vi "Trajectory Loading v2.vi"(6 "PID Cluster":T6={"L1 to L4 PID Cluster"={"L1 PID Gains"={"Kp"=0.005, "Kd"=0.5, "Ki"=0.0005}, "L2 PID Gains"={"Kp"=0.01, "Kd"=1.0, "Ki"=0.005}, "L3 PID Gains"={"Kp"=0.05, "Kd"=1.0, "Ki"=0.0005}, "L4 PID Gains"={"Kp"=0.1, "Kd"=0.1, "Ki"=0.0005}}, "Stage PID Cluster"={"Stage Z PID"={"Kp"=0.0005, "Kd"=0.001, "Ki"=0.0}, "Stage Y PID"={"Kp"=0.0003, "Kd"=0.01, "Ki"=0.0}, "Stage X PID"={"Kp"=0.0003, "Kd"=0.01, "Ki"=0.0}}, "OCT Z PID Gains"={"Kp"=0.0003, "Kd"=0.0001, "Ki"=0.01}}, 7 "Robot In":i32, 8 "error in":errorcluster, 10 "Prev Posit Cluster":T5={"Prev L1 to L4 Posit"=[-0.5319, -0.035669172703475985, -2.0566170657346783, 0.9099264705882353], "Prev Stage Posit"=[6.002553885707208, 5.996566124542428, 5.995469940427586], "Prev OCT Z Posit"=-0.0}, 11 "FPGA VI Reference In":refnum<k20>) -> (0 "Eye Model Cluster":T3={"X Grid"=[], "Y Grid"=[], "Za_true Surf"=[], "Iris Center"=[0.0, 5.0, 0.0], "Zp_true Surf"=[], "Pinv"=[[1.0, 0.0], [0.0, 1.0]], "za_true"=0.0, "za_work"=0.0, "zp_work"=0.0, "zp_true"=0.0}, 1 "Trajectory Cluster":T1, 2 "Last Posit Cluster":T4={"Last L1 to L4 Posit"=[0.0, 0.0, 0.0, 0.0], "Last Stage Posit"=[6.0, 6.0, 6.0], "Last OCT Z Posit"=0.0}, 3 "FPGA VI Reference Out":refnum<k20>, 4 "error out":errorcluster, 5 "First Trk Pt":dbl[](array[numeric]))   [LabVIEW 2016]
uses:
  Subsystems/Global Variables.vi
  <vilib>/Platform/TimedLoop/XDataNode/wakeup.ctl
  <vilib>/Platform/TimedLoop/XDataNode/XDNodeRunTimeDep.lvlib
  <vilib>/Platform/TimedLoop/XDataNode/nitl_modes.ctl
  <vilib>/Platform/TimedLoop/XDataNode/timing_clust.ctl
  <vilib>/platform/TimedLoop/XDataNode/XDataNode.xnode
  <vilib>/Analysis/Matrix/Datatypes/RealMatrix.ctl
  <vilib>/Analysis/Matrix/NI_Matrix.lvlib
panel:
  out "In Servo Loop":bool
  out "Loading Finished":bool
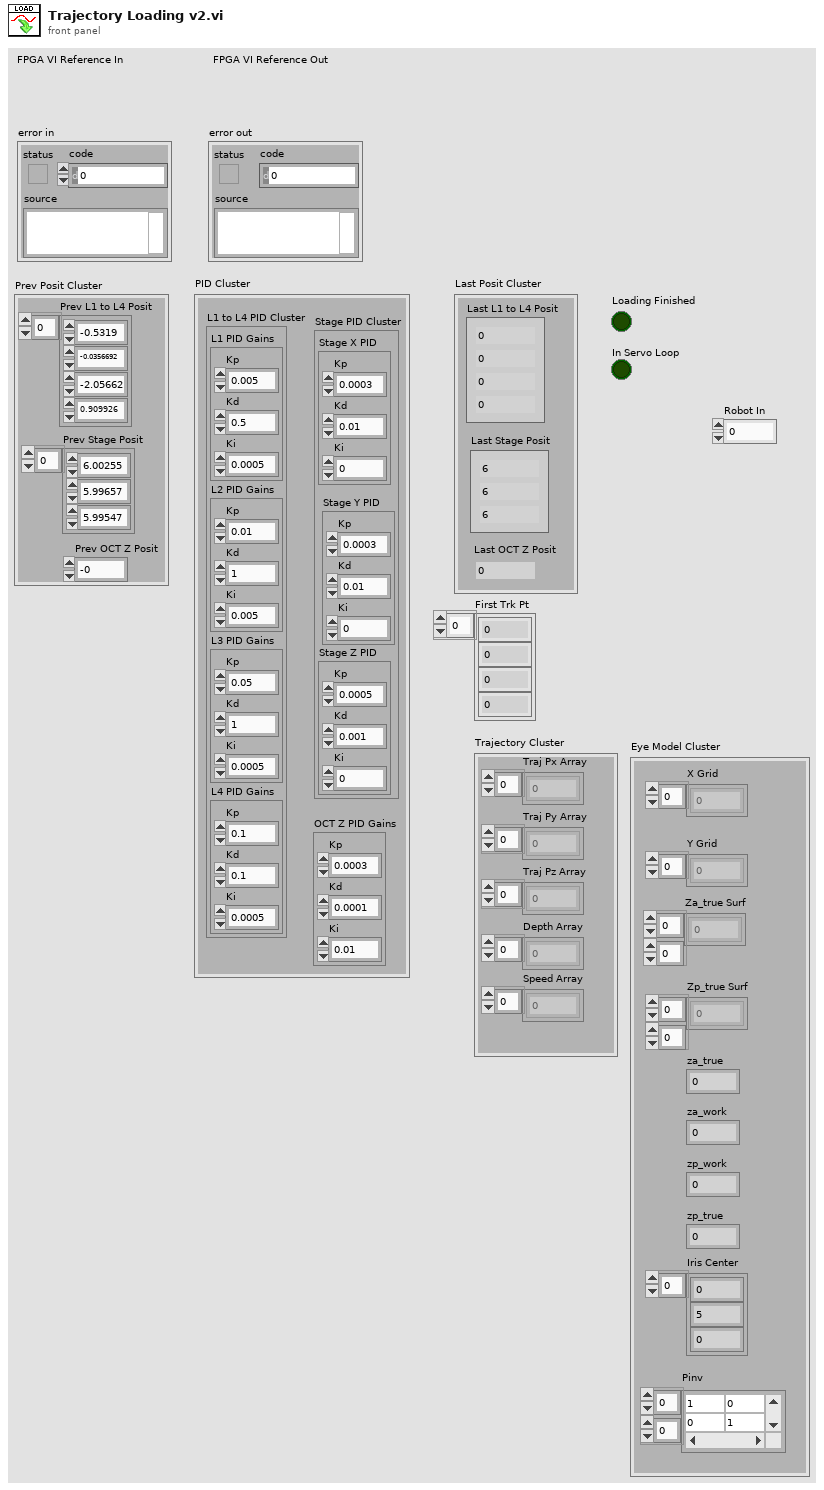
[diagram p1: front panel]
types:
  T1 = cluster{"Traj Px Array":dbl[], "Traj Py Array":dbl[], "Traj Pz Array":dbl[], "Speed Array":dbl[], "Depth Array":dbl[]}
  T2 = typedef "NI_Matrix.lvlib/RealMatrix.ctl" = dbl[][]
  T3 = cluster{"X Grid":dbl[], "Y Grid":dbl[], "Za_true Surf":dbl[][], "Iris Center":dbl[], "Zp_true Surf":dbl[][], "Pinv":T2, "za_true":dbl, "za_work":dbl, "zp_work":dbl, "zp_true":dbl}
  T4 = cluster{"Last L1 to L4 Posit":dbl[], "Last Stage Posit":dbl[], "Last OCT Z Posit":dbl}
  T5 = cluster{"Prev L1 to L4 Posit":dbl[], "Prev Stage Posit":dbl[], "Prev OCT Z Posit":dbl}
  T6 = cluster{"L1 to L4 PID Cluster":cluster{"L1 PID Gains":cluster{"Kp":dbl, "Kd":dbl, "Ki":dbl}, "L2 PID Gains":cluster{"Kp":dbl, "Kd":dbl, "Ki":dbl}, "L3 PID Gains":cluster{"Kp":dbl, "Kd":dbl, "Ki":dbl}, "L4 PID Gains":cluster{"Kp":dbl, "Kd":dbl, "Ki":dbl}}, "Stage PID Cluster":cluster{"Stage Z PID":cluster{"Kp":dbl, "Kd":dbl, "Ki":dbl}, "Stage Y PID":cluster{"Kp":dbl, "Kd":dbl, "Ki":dbl}, "Stage X PID":cluster{"Kp":dbl, "Kd":dbl, "Ki":dbl}}, "OCT Z PID Gains":cluster{"Kp":dbl, "Kd":dbl, "Ki":dbl}}
  T7 = typedef "XDNodeRunTimeDep.lvlib/timing_clust.ctl" = cluster{"Expected End [f-1]":u64, "Actual End [f-1]":u64, "Finished Late? [f-1]":bool, "Expected End [i-1]":u64, "Actual End [i-1]":u64, "Finished Late? [i-1]":bool, "Expected Start [i]":u64, "Actual Start [i]":u64, "Expected Start [f]":u64, "Actual Start [f]":u64, "Source Name":string, "Structure Name":string, "Period":i64, "Deadline":i64, "Offset":i64, "Start":i64, "Priority":i32, "Timeout":i32, "Mode":T8, "Wakeup Reason":T9, "Error":errorcluster, "Source Type":string, "Secondary Source Type":string, "Global End Time":u64, "Global Start Time":u64, "Frame Duration":u64, "Iteration Duration":u64, "Assigned CPU":i32, "I/O Scan Engine Mode":u32}
  T8 = typedef "XDNodeRunTimeDep.lvlib/nitl_modes.ctl" = enum32{"No Change", "Process missed periods, maintain original phase", "Discard missed periods, maintain original phase", "Process missed periods, ignore original phase", "Discard missed periods, ignore original phase"}
  T9 = typedef "XDNodeRunTimeDep.lvlib/wakeup.ctl" = enum32{"Normal", "Aborted", "Asynchronous wakeup", "Timing source error", "Timed loop error", "Timeout"}
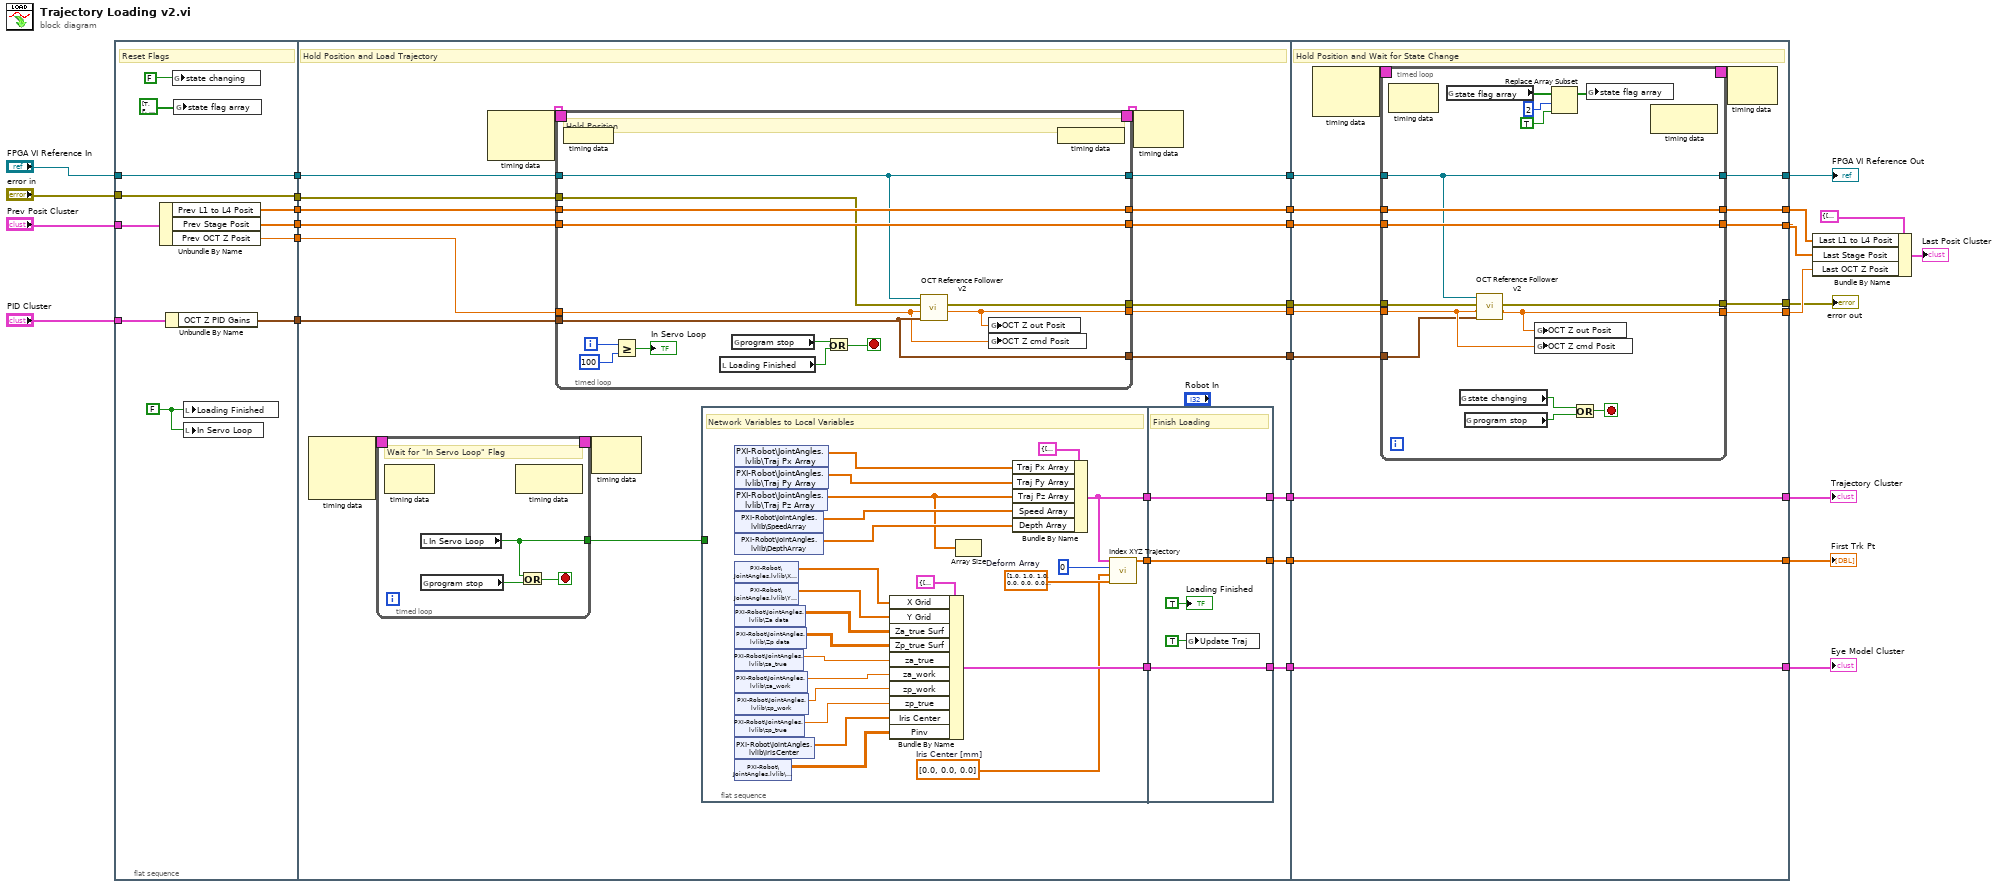
[diagram p0: block diagram]
diagram:
  n1 = flat-sequence {
    tunnel: [w38] -> w29
    tunnel: "FPGA VI Reference In" -> [w38]
    tunnel: [w37] -> w27
    tunnel: "error in" -> [w37]
    tunnel: "Prev Posit Cluster" -> [w36]
    tunnel: "PID Cluster" -> [w35]
    tunnel: [w34] -> w23
    tunnel: [w33] -> w22
    tunnel: [w32] -> w21
    tunnel: [w30] -> w20
    tunnel: w29 -> [w50]
    tunnel: w27 -> [w47]
    tunnel: w23 -> [w49]
    tunnel: w22 -> [w46]
    tunnel: w21 -> [w45]
    tunnel: w20 -> [w48]
    tunnel: [w63] -> w11
    tunnel: [w62] -> w10
    tunnel: [w61] -> w9
    tunnel: [w60] -> w8
    tunnel: [w59] -> w7
    tunnel: [w58] -> w6
    tunnel: [w41] -> w5
    tunnel: [w44] -> w4
    tunnel: [w42] -> w3
    tunnel: w11 -> [w130]
    tunnel: [w129] -> w1
    tunnel: w10 -> [w128]
    tunnel: w9 -> [w127]
    tunnel: w8 -> [w126]
    tunnel: w7 -> [w125]
    tunnel: [w124] -> w18
    tunnel: [w123] -> w17
    tunnel: [w122] -> w16
    tunnel: [w121] -> w14
    tunnel: [w118] -> w12
    tunnel: w6 -> [w120]
    tunnel: [w120] -> w13
    tunnel: w5 -> [w119]
    tunnel: w4 -> [w118]
    tunnel: [w117] -> w2
    tunnel: w3 -> [w117]
    frame #0 {
      w31 = FALSE ("Loading Finished")
      # "Reset Flags"
      n2 = Unbundle By Name(w36) -> ("Prev L1 to L4 Posit"=w34:dbl[], "Prev Stage Posit"=w33:dbl[], "Prev OCT Z Posit"=w32:dbl)
      n3 = Unbundle By Name(w35) -> ("OCT Z PID Gains"=w30:cluster{"Kp":dbl, "Kd":dbl, "Ki":dbl})
      n4 = global write "Global Variables.vi" "state changing"(FALSE ("state changing")) -> ()
      n5 = global write "Global Variables.vi" "state flag array"(bool[] [TRUE, FALSE, FALSE, FALSE, FALSE, FALSE, FALSE, FALSE, FALSE] ("state flag array")) -> ()
      n6 = local write "Loading Finished"(w31) -> ()
      n7 = local write "In Servo Loop"(w31) -> ()
    }
    frame #1 {
      # "Hold Position and Load Trajectory"
      n8 = node-c288() -> (w53:T7)  [unwired: 3 in]
      n9 = timed-loop {
        timing: w53 -> [_]
        timing-out: [_] -> w52
        tunnel: [w65] -> w51
        stop <- w66 stop-if-true
        # "Wait for \"In Servo Loop\" Flag"
        n10 = node-c288() -> ()  [unwired: 1 in, 1 out]
        n11 = local read "In Servo Loop"() -> (w65:bool)
        n12 = global read "Global Variables.vi" "program stop"() -> (w64:bool)
        n13 = node-c288() -> ()  [unwired: 1 in, 1 out]
        n14 = Or(x=w65, y=w64) -> (x .or. y?=w66:bool)
      }
      n15 = node-c288() -> (w57:T7)  [unwired: 2 in]
      n16 = timed-loop {
        timing: w57 -> [_]
        timing-out: [_] -> w56
        tunnel: w49 -> [w105]
        tunnel: w46 -> [w106]
        tunnel: w47 -> [w102]
        tunnel: w50 -> [w101]
        tunnel: w45 -> [w103]
        tunnel: w48 -> [w104]
        tunnel: [w105] -> w62
        tunnel: [w106] -> w61
        tunnel: [w99] -> w60
        tunnel: [w101] -> w63
        tunnel: [w100] -> w41
        tunnel: [w104] -> w59
        i -> [w109]
        stop <- w112 stop-if-true
        # "Hold Position"
        n17 = node-c288 ("Output Node")() -> ()  [unwired: 1 in]
        n18 = Greater Or Equal?(x=w109, y=100) -> (x >= y?=→"In Servo Loop":bool)
        n19 = local read "Loading Finished"() -> (w111:bool)
        n20 = global read "Global Variables.vi" "program stop"() -> (w110:bool)
        n21 = Or(x=w110, y=w111) -> (x .or. y?=w112:bool)
        n22 = call "OCT Reference Follower v2.vi"("OCT Z PID Gains"=w104, "OCT  Z cmd Posit [mm]"=w103, "error in"=w102, "FPGA VI Reference In"=w101) -> ("OCT  Z out Posit [mm]"=w99:dbl, "error out"=w100:errorcluster)  [unwired: 5 in, 1 out]
        n23 = global write "Global Variables.vi" "OCT Z out Posit"(w99) -> ()
        n24 = global write "Global Variables.vi" "OCT Z cmd Posit"(w103) -> ()
        n25 = node-c288() -> ()  [unwired: 1 out]
      }
      n26 = node-c288(w52) -> ()  [unwired: 1 out]
      n27 = flat-sequence {
        tunnel: [w79] -> w55
        tunnel: [w80] -> w54
        tunnel: w51 -> [_]
        tunnel: [w78] -> w43
        tunnel: [w97] -> w58
        tunnel: w55 -> [w96]
        tunnel: w54 -> [w97]
        tunnel: [w96] -> w44
        tunnel: [w95] -> w42
        tunnel: w43 -> [w95]
        frame #0 {
          w75 = dbl[] [0.0, 0.0, 0.0]  # Iris Center [mm]
          w76 = dbl[] [1.0, 1.0, 1.0, 0.0, 0.0, 0.0, 0.0, 0.0, 0.0]  # Deform Array
          # "Network Variables to Local Variables"
          n28 = shared-variable "PXI-Robot\\JointAngles.lvlib\\Traj Px Array"() -> (w73:dbl[])  [unwired: 1 in, 1 out]
          n29 = shared-variable "PXI-Robot\\JointAngles.lvlib\\Traj Py Array"() -> (w72:dbl[])  [unwired: 1 in, 1 out]
          n30 = shared-variable "PXI-Robot\\JointAngles.lvlib\\Traj Pz Array"() -> (w71:dbl[])  [unwired: 1 in, 1 out]
          n31 = shared-variable "PXI-Robot\\JointAngles.lvlib\\SpeedArray"() -> (w82:dbl[])  [unwired: 1 in, 1 out]
          n32 = shared-variable "PXI-Robot\\JointAngles.lvlib\\DepthArray"() -> (w81:dbl[])  [unwired: 1 in, 1 out]
          n33 = shared-variable "PXI-Robot\\JointAngles.lvlib\\X grid"() -> (w93:dbl[])  [unwired: 1 in, 1 out]
          n34 = shared-variable "PXI-Robot\\JointAngles.lvlib\\Y grid"() -> (w92:dbl[])  [unwired: 1 in, 1 out]
          n35 = shared-variable "PXI-Robot\\JointAngles.lvlib\\Za data"() -> (w91:dbl[][])  [unwired: 1 in, 1 out]
          n36 = shared-variable "PXI-Robot\\JointAngles.lvlib\\Zp data"() -> (w89:dbl[][])  [unwired: 1 in, 1 out]
          n37 = shared-variable "PXI-Robot\\JointAngles.lvlib\\za_true"() -> (w84:dbl)  [unwired: 1 in, 1 out]
          n38 = shared-variable "PXI-Robot\\JointAngles.lvlib\\za_work"() -> (w85:dbl)  [unwired: 1 in, 1 out]
          n39 = shared-variable "PXI-Robot\\JointAngles.lvlib\\zp_work"() -> (w86:dbl)  [unwired: 1 in, 1 out]
          n40 = shared-variable "PXI-Robot\\JointAngles.lvlib\\zp_true"() -> (w87:dbl)  [unwired: 1 in, 1 out]
          n41 = shared-variable "PXI-Robot\\JointAngles.lvlib\\IrisCenter"() -> (w74:dbl[])  [unwired: 1 in, 1 out]
          n42 = shared-variable "PXI-Robot\\JointAngles.lvlib\\Pinv"() -> (w88:T2)  [unwired: 1 in, 1 out]
          n43 = Bundle By Name(cluster=T3 {"X Grid"=[], "Y Grid"=[], "Za_true Surf"=[], "Iris Center"=[], "Zp_true Surf"=[], "Pinv"=[], "za_true"=0.0, "za_work"=0.0, "zp_work"=0.0, "zp_true"=0.0} ("Eye Model Cluster"), "X Grid"=w93, "Y Grid"=w92, "Za_true Surf"=w91, "Zp_true Surf"=w89, "za_true"=w84, "za_work"=w85, "zp_work"=w86, "zp_true"=w87, "Iris Center"=w74, "Pinv"=w88) -> (w80:T3)
          n44 = Array Size(array=w71) -> ()  [unwired: 1 out]
          n45 = Bundle By Name(cluster=T1 {"Traj Px Array"=[], "Traj Py Array"=[], "Traj Pz Array"=[], "Speed Array"=[], "Depth Array"=[]} ("Trajectory Cluster"), "Traj Px Array"=w73, "Traj Py Array"=w72, "Traj Pz Array"=w71, "Speed Array"=w82, "Depth Array"=w81) -> (w79:T1)
          n46 = call "Index XYZ Trajectory.vi"("Deform Array"=w76, "Pivot Pt"=w75, "Index"=0 ("index"), "Trajectory Cluster"=w79) -> ("Indexed XYZ Posit"=w78:dbl[])  [unwired: 6 in, 1 out]
        }
        frame #1 {
          # "Finish Loading"
          n47 = global write "Global Variables.vi" "Update Traj"(TRUE ("Update Traj")) -> ()
          "Loading Finished" <- TRUE ("Loading Finished")
        }
      }
      n48 = node-c288(w56) -> ()  [unwired: 1 out]
    }
    frame #2 {
      # "Hold Position and Wait for State Change"
      n49 = node-c288() -> (w132:T7)  [unwired: 2 in]
      n50 = timed-loop {
        timing: w132 -> [_]
        timing-out: [_] -> w131
        tunnel: w130 -> [w138]
        tunnel: [w134] -> w129
        tunnel: w128 -> [w139]
        tunnel: w127 -> [w140]
        tunnel: w126 -> [w136]
        tunnel: w125 -> [w135]
        tunnel: [w139] -> w124
        tunnel: [w140] -> w123
        tunnel: [w133] -> w122
        tunnel: [w138] -> w121
        tunnel: w119 -> [w137]
        stop <- w147 stop-if-true
        n51 = node-c288() -> ()  [unwired: 1 in, 1 out]
        n52 = global read "Global Variables.vi" "state flag array"() -> (w144:bool[])
        n53 = global read "Global Variables.vi" "state changing"() -> (w146:bool)
        n54 = global read "Global Variables.vi" "program stop"() -> (w145:bool)
        n55 = call "OCT Reference Follower v2.vi"("OCT Z PID Gains"=w135, "OCT  Z cmd Posit [mm]"=w136, "error in"=w137, "FPGA VI Reference In"=w138) -> ("OCT  Z out Posit [mm]"=w133:dbl, "error out"=w134:errorcluster)  [unwired: 5 in, 1 out]
        n56 = global write "Global Variables.vi" "OCT Z out Posit"(w133) -> ()
        n57 = global write "Global Variables.vi" "OCT Z cmd Posit"(w136) -> ()
        n58 = Replace Array Subset(array=w144, new element=TRUE ("new element/subarray"), index=2) -> (w143:bool[])
        n59 = Or(x=w146, y=w145) -> (x .or. y?=w147:bool)
        n60 = global write "Global Variables.vi" "state flag array"(w143) -> ()
        n61 = node-c288() -> ()  [unwired: 1 in, 1 out]
      }
      n62 = node-c288(w131) -> ()  [unwired: 1 out]
    }
  }
  n63 = Bundle By Name(cluster=T4 {"Last L1 to L4 Posit"=[0.0, 0.0, 0.0, 0.0], "Last Stage Posit"=[6.0, 6.0, 6.0], "Last OCT Z Posit"=0.0} ("Last Posit Cluster 2"), "Last L1 to L4 Posit"=w18, "Last Stage Posit"=w17, "Last OCT Z Posit"=w16) -> (→"Last Posit Cluster":T4)
  "FPGA VI Reference Out" <- w14
  "error out" <- w1
  "First Trk Pt" <- w2
  "Eye Model Cluster" <- w13
  "Trajectory Cluster" <- w12
